vi "ISX3_Disconnect.vi"(2 "FT_Handle":u32) -> ()   [LabVIEW 2012, in "Sciospec ISX3 Impedance Analyzer.lvlib"]
uses:
  Sciospec ISX3 Impedance Analyzer.lvlib
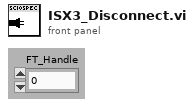
[diagram p1: front panel]
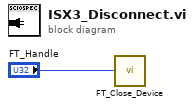
[diagram p0: block diagram]
diagram:
  n1 = call "FT_Close_Device.vi"("Handle"="FT_Handle") -> ()  [unwired: 1 out]
